vi "test find files.vi"() -> ()   [LabVIEW 2014]
uses:
  <vilib>/FTP/NI_FTP.lvlib
  <vilib>/FTP/ftp2.llb/FTP File Info.ctl
panel:
  in  "local path":path
  in  "file specifications":T1(array[cluster])
  out "dir list":T2[](array[typedef])
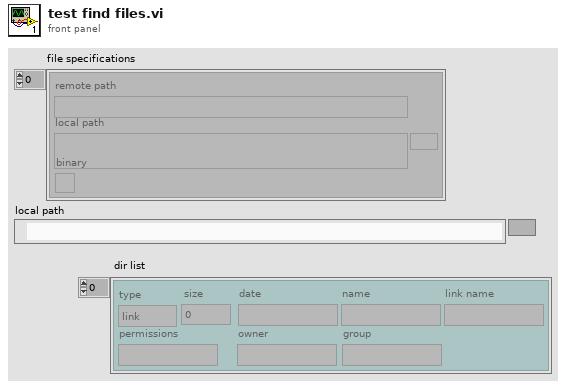
[diagram p1: front panel]
types:
  T1 = cluster{"remote path":string, "local path":path, "binary":bool}[]
  T2 = typedef "NI_FTP.lvlib/FTP File Info.ctl" = cluster{"type":enum16{"unknown", "file", "dir", "link"}, "permissions":string, "owner":string, "group":string, "size":i32, "date":string, "name":string, "link name":string}
  T3 = typedef "NI_FTP.lvlib/FTP Session.ctl" = refnum<k5>
  T4 = cluster{"remote path":string, "local path":path, "binary":bool}
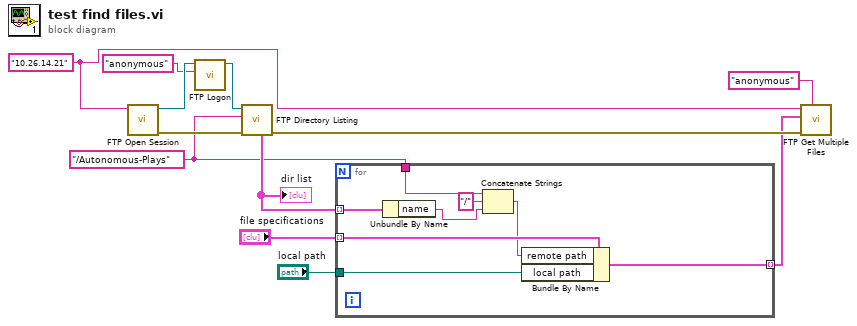
[diagram p0: block diagram]
diagram:
  w3 = "/Autonomous-Plays" ("directory path")
  w7 = "10.26.14.21" ("host")
  n1 = call <vilib>:"FTP Open Session.vi"("address"=w7) -> ("error out"=w12:errorcluster, "ftp session"=w11:T3)  [unwired: 7 in, 2 out]
  n2 = call <vilib>:"FTP Logon.vi"("user"="anonymous", "ftp session"=w11) -> ("ftp session out"=w9:T3)  [unwired: 6 in, 3 out]
  n3 = call <vilib>:"FTP Directory Listing.vi"("error in (no error)"=w12, "directory path"=w3, "ftp session"=w9) -> ("error out"=w6:errorcluster, "dir list"=w5:T2[])  [unwired: 4 in, 3 out]
  "dir list" <- w5
  n4 = for {
    tunnel: w5 -> [w19] mode=indexing
    tunnel: "file specifications" -> [w18] mode=indexing
    tunnel: w3 -> [w20]
    tunnel: "local path" -> [w17]
    tunnel: [w13] -> w1 mode=indexing
    n5 = Unbundle By Name(w19) -> ("name"=w15:string)
    n6 = Concatenate Strings(w20, "/" ("string"), w15) -> (w14:string)
    n7 = Bundle By Name(cluster=w18, "remote path"=w14, "local path"=w17) -> (w13:T4)
  }
  n8 = call <vilib>:"FTP Get Multiple Files.vi"("user"="anonymous", "error in (no error)"=w6, "file specifications"=w1, "host"=w7) -> ()  [unwired: 6 in, 2 out]
